vi "Convert Data to ChangeDTCCount.vi"(8 "error in (no error)":errorcluster, 11 "Data":T1[](array[typedef]) {"payload" format="%x"; "timestamp" format="%<%.7X\n%x>T"; "type" items=["CAN Data"=0, "CAN Remote"=1, "CAN Bus Error"=2, "J1939 Data"=192, "Delay"=224, "Log Trigger"=225, "Start Trigger"=226]; "identifier" format="%x"}) -> (0 "error out":errorcluster, 3 "ChangeDTCCount":u16)   [LabVIEW 2015, in "GMLAN.lvlib"]
uses:
  GMLAN.lvlib
  <vilib>/xnet/xnet.llb/XNET Frame CAN.ctl
  <vilib>/xnet/xnet.llb/XNET Frame Type CAN.ctl
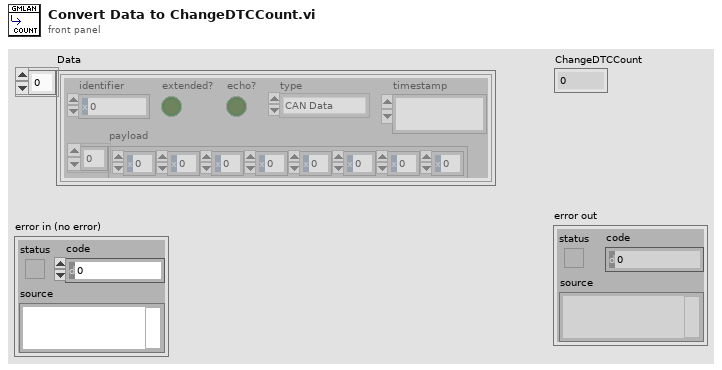
[diagram p1: front panel]
types:
  T1 = typedef "XNET Frame CAN.ctl" = cluster{"timestamp":timestamp, "payload":u8[], "identifier":u32, "type":T2, "extended?":bool, "echo?":bool}
  T2 = typedef "XNET Frame Type CAN.ctl" = u8
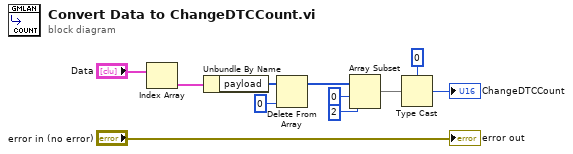
[diagram p0: block diagram]
diagram:
  n1 = Index Array(array="Data") -> (element=w3:T1)  [unwired: 1 in]
  n2 = Unbundle By Name(w3) -> ("payload"=w11:u8[])
  n3 = Delete From Array(array=w11, index=0) -> (array with subset deleted=w5:u8[])  [unwired: 1 in, 1 out]
  n4 = Array Subset(array=w5, index=0, length=2) -> (w7:u8[])
  n5 = Type Cast(type=u16 0 ("length"), x=w7) -> (*(type *) &x=→"ChangeDTCCount":u16)
  "error out" <- "error in (no error)"
